vi "current pulse2.vi"() -> ()   [LabVIEW 2018]
doc: "Configures a sweep and takes voltage and current readings at each point."
uses:
  <instrlib>/Keithley 2450/Public/Data/Read (Multiple Points).vi
  <instrlib>/Keithley 2450/Keithley 2450.lvlib
panel:
  in  "Current":dbl
  in  "Count":dbl
  in  "Delay (0) in Sec":dbl=0.001
  in  "VISA resource name":refnum<visa-resource-name>
  out "Waveform Graph":dbl[][](graph)
  in  "Limit  Level (0.1)":dbl=0.1
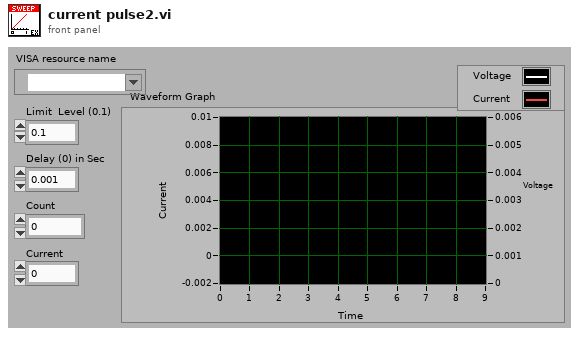
[diagram p1: front panel]
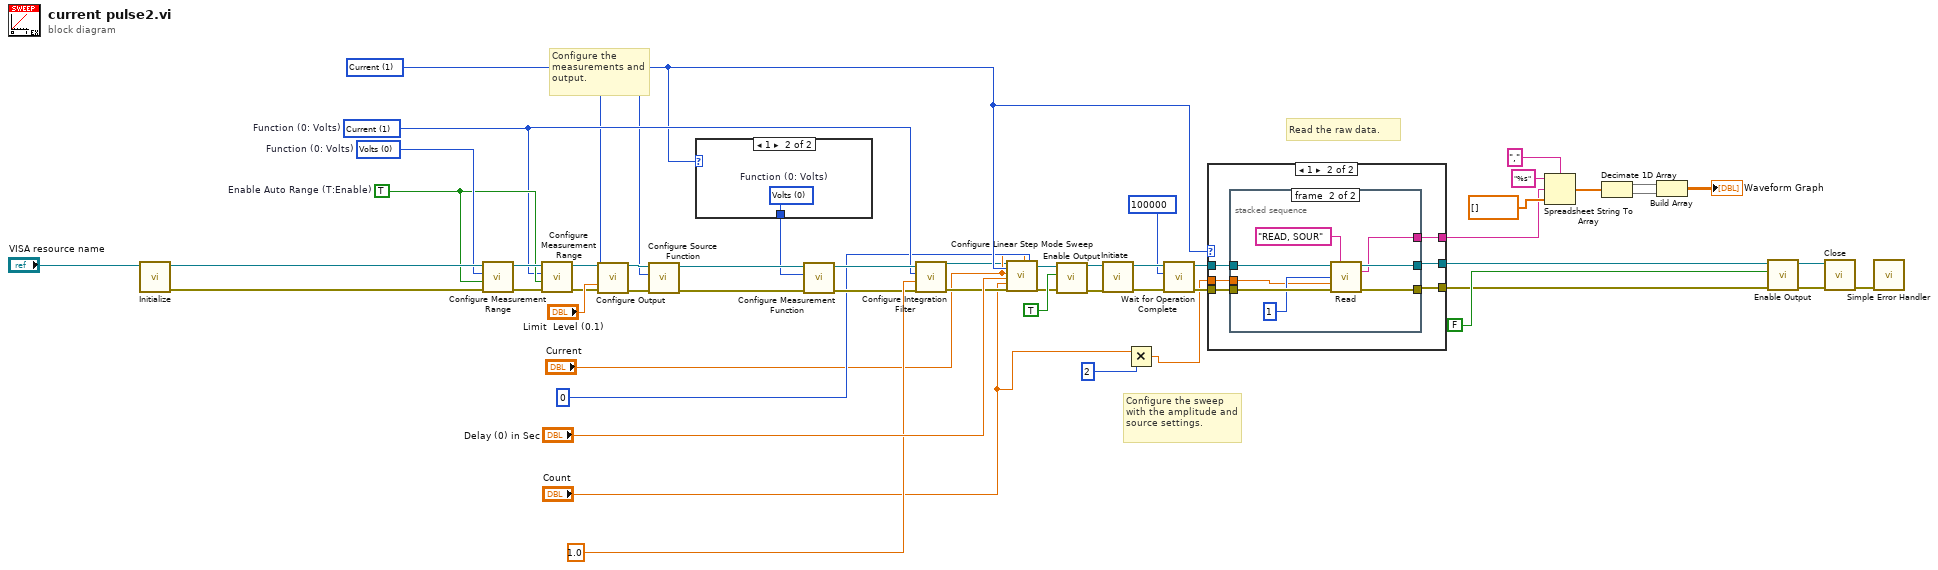
[diagram p0: block diagram]
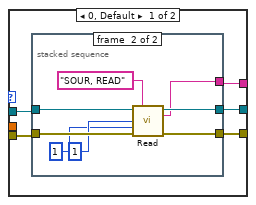
[diagram p2: hidden frame]
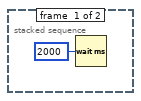
[diagram p3: hidden frame]
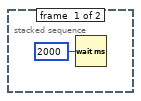
[diagram p4: hidden frame]
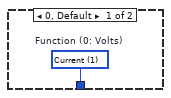
[diagram p5: hidden frame]
diagram:
  w13 = u16 1 items=["Voltage", "Current"] ("Source Mode  (0: Voltage)")
  w41 = TRUE  # Enable Auto Range (T:Enable)
  w15 = u16 1 items=["Volts", "Current", "Resistance"]  # Function (0: Volts)
  w42 = u16 0 items=["Volts", "Current", "Resistance"]  # Function (0: Volts)
  # "Read the raw data."
  # "Configure the sweep with the amplitude and source settings."
  # "Configure the measurements and output."
  n1 = call <instrlib>:"Initialize.vi"("VISA resource name"="VISA resource name") -> ("error out"=w51:errorcluster, "VISA resource name out"=w52:refnum<visa-resource-name>)  [unwired: 9 in]
  n2 = call <instrlib>:"Configure Measurement Range.vi"("error in (no error)"=w51, "Enable Auto Range (T:Enable)"=w41, "Function (0: Volts)"=w42, "VISA resource name"=w52) -> ("error out"=w50:errorcluster, "VISA resource name out"=w49:refnum<visa-resource-name>)  [unwired: 6 in]
  n3 = call <instrlib>:"Configure Measurement Range.vi"("error in (no error)"=w50, "Enable Auto Range (T:Enable)"=w41, "Function (0: Volts)"=w15, "VISA resource name"=w49) -> ("error out"=w38:errorcluster, "VISA resource name out"=w39:refnum<visa-resource-name>)  [unwired: 6 in]
  n4 = call <instrlib>:"Configure Output.vi"("VISA resource name"=w39, "Source Mode  (0: Voltage)"=w13, "Source Limit Level (0.1)"="Limit  Level (0.1)", "error in (no error)"=w38) -> ("VISA resource name out"=w36:refnum<visa-resource-name>, "error out"=w37:errorcluster)  [unwired: 10 in]
  n5 = call <instrlib>:"Configure Source Function.vi"("error in (no error)"=w37, "Function (0: Volts)"=w13, "VISA resource name"=w36) -> ("error out"=w18:errorcluster, "VISA resource name out"=w19:refnum<visa-resource-name>)  [unwired: 7 in]
  n6 = case shown="1" w13 {
    tunnel: [w53 w54] -> w14
    frame 0, Default {
      w53 = u16 1 items=["Volts", "Current", "Resistance"]  # Function (0: Volts)
    }
    frame 1 {
      w54 = u16 0 items=["Volts", "Current", "Resistance"]  # Function (0: Volts)
    }
  }
  n7 = call <instrlib>:"Configure Measurement Function.vi"("error in (no error)"=w18, "Function (0: Volts)"=w14, "VISA resource name"=w19) -> ("error out"=w17:errorcluster, "VISA resource name out"=w16:refnum<visa-resource-name>)  [unwired: 7 in]
  n8 = call <instrlib>:"Configure Integration Filter.vi"("error in (no error)"=w17, "Measurement Speed (1 PLC)"=1.0, "Function (0: Volts)"=w15, "VISA resource name"=w16) -> ("error out"=w22:errorcluster, "VISA resource name out"=w4:refnum<visa-resource-name>)  [unwired: 6 in]
  n9 = call <instrlib>:"Configure Linear Step Mode Sweep.vi"("VISA resource name"=w4, "Source Mode  (0: Voltage)"=w13, "Stop"="Current", "Delay (0)"="Delay (0) in Sec", "Count (1)"="Count", "error in (no error)"=w22, "Step"="Current", "Start"=0) -> ("VISA resource name out"=w34:refnum<visa-resource-name>, "error out"=w33:errorcluster)  [unwired: 10 in]
  n10 = call <instrlib>:"Enable Output.vi"("error in (no error)"=w33, "Enable Output (T: Enable)"=TRUE, "VISA resource name"=w34) -> ("error out"=w31:errorcluster, "VISA resource name out"=w32:refnum<visa-resource-name>)  [unwired: 7 in]
  n11 = call <instrlib>:"Initiate.vi"("error in (no error)"=w31, "VISA resource name"=w32) -> ("error out"=w23:errorcluster, "VISA resource name out"=w24:refnum<visa-resource-name>)  [unwired: 8 in]
  n12 = Multiply(x="Count", y=2) -> (x*y=w1:dbl)
  n13 = call <instrlib>:"Wait for Operation Complete.vi"("error in (no error)"=w23, "Timeout (10000 ms)"=100000, "VISA resource name"=w24) -> ("error out"=w11:errorcluster, "VISA resource name out"=w12:refnum<visa-resource-name>)  [unwired: 7 in]
  n14 = case shown="1" w13 {
    tunnel: w12 -> [w59 w74]
    tunnel: w11 -> [w58 w73]
    tunnel: [w57 w72] -> w10
    tunnel: [w56 w71] -> w9
    tunnel: [w55 w70] -> w8
    tunnel: w1 -> [_ w69]
    frame 0, Default {
      n15 = stacked-sequence {
        tunnel: [_ w68] -> w57
        tunnel: [_ w67] -> w56
        tunnel: w59 -> [_ w65]
        tunnel: w58 -> [_ w64]
        tunnel: [_ w63] -> w55
        frame #0 {
          n16 = Wait (ms)(milliseconds to wait=u32 2000) -> ()  [unwired: 1 out]
        }
        frame #1 {
          n17 = call-poly <instrlib>:"Read.vi"("VISA resource name"=w65, "Buffer Elements"="SOUR, READ", "Start Index (1)"=1, "End Index (1)"=1, "error in (no error)"=w64) -> ("VISA resource name out"=w68:refnum<visa-resource-name>, "Data out"=w63:string, "error out"=w67:errorcluster)  [unwired: 8 in]
        }
      }
    }
    frame 1 {
      n18 = stacked-sequence {
        tunnel: [_ w83] -> w72
        tunnel: [_ w82] -> w71
        tunnel: w74 -> [_ w80]
        tunnel: w73 -> [_ w79]
        tunnel: [_ w78] -> w70
        tunnel: w69 -> [_ w76]
        frame #0 {
          n19 = Wait (ms)(milliseconds to wait=u32 2000) -> ()  [unwired: 1 out]
        }
        frame #1 {
          n20 = call-poly <instrlib>:"Read.vi"("VISA resource name"=w80, "Buffer Elements"="READ, SOUR", "Start Index (1)"=1, "End Index (1)"=w76, "error in (no error)"=w79) -> ("VISA resource name out"=w83:refnum<visa-resource-name>, "Data out"=w78:string, "error out"=w82:errorcluster)  [unwired: 8 in]
        }
      }
    }
  }
  n21 = Spreadsheet String To Array(delimiter (Tab)=",", format string="%s", spreadsheet string=w8, array type (2D Dbl)=dbl[] []) -> (array=w27:dbl[])
  n22 = Decimate 1D Array(w27) -> (w26:dbl[], w25:dbl[])
  n23 = Build Array(w26, w25) -> (→"Waveform Graph":dbl[][])
  n24 = call <instrlib>:"Enable Output.vi"("error in (no error)"=w9, "Enable Output (T: Enable)"=FALSE, "VISA resource name"=w10) -> ("error out"=w45:errorcluster, "VISA resource name out"=w46:refnum<visa-resource-name>)  [unwired: 7 in]
  n25 = call <instrlib>:"Close.vi"("error in (no error)"=w45, "VISA resource name"=w46) -> ("error out"=w47:errorcluster)  [unwired: 9 in]
  n26 = call <vilib>:"Simple Error Handler.vi"("error in (no error)"=w47) -> ()  [unwired: 4 in, 5 out]
